vi "Init Controls.vi"(7 "connected":bool, 8 "Fehler (Eingang, kein Fehler)":errorcluster, 10 "Cluster Refernz Cluster":T1, 11 "Info Cluster":T2) -> (0 "Fehler (Ausgang)":errorcluster, 6 "connected out":bool)   [LabVIEW 2020, in "Linearisierung v2.lvlib" / "Gasteiler.lvlib" / "HovaCAL_Interface.lvlib" / "Helper.lvlib"]
uses:
  Helper.lvlib
  Controls/Info Cluster.ctl
  Controls/Controls.lvlib
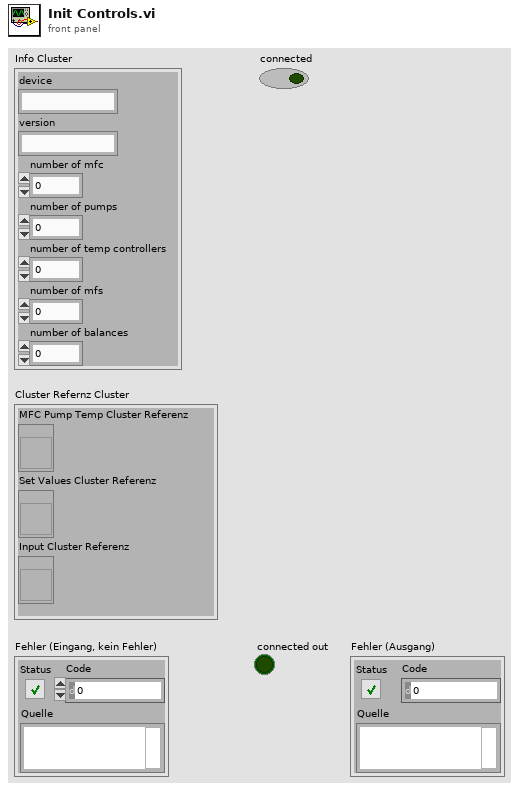
[diagram p1: front panel]
types:
  T1 = cluster{"MFC Pump Temp Cluster Referenz":refnum<vi>, "Set Values Cluster Referenz":refnum<vi>, "Input Cluster Referenz":refnum<vi>}
  T2 = typedef "Linearisierung v2.lvlib/Gasteiler.lvlib/HovaCAL_Interface.lvlib/Controls.lvlib/Info Cluster.ctl" = cluster{"device":string, "version":string, "number of mfc":i32, "number of pumps":i32, "number of temp controllers":i32, "number of mfs":i32, "number of balances":i32}
  T3 = enum8{"Enabled", "Disabled", "Disabled and Grayed Out"}
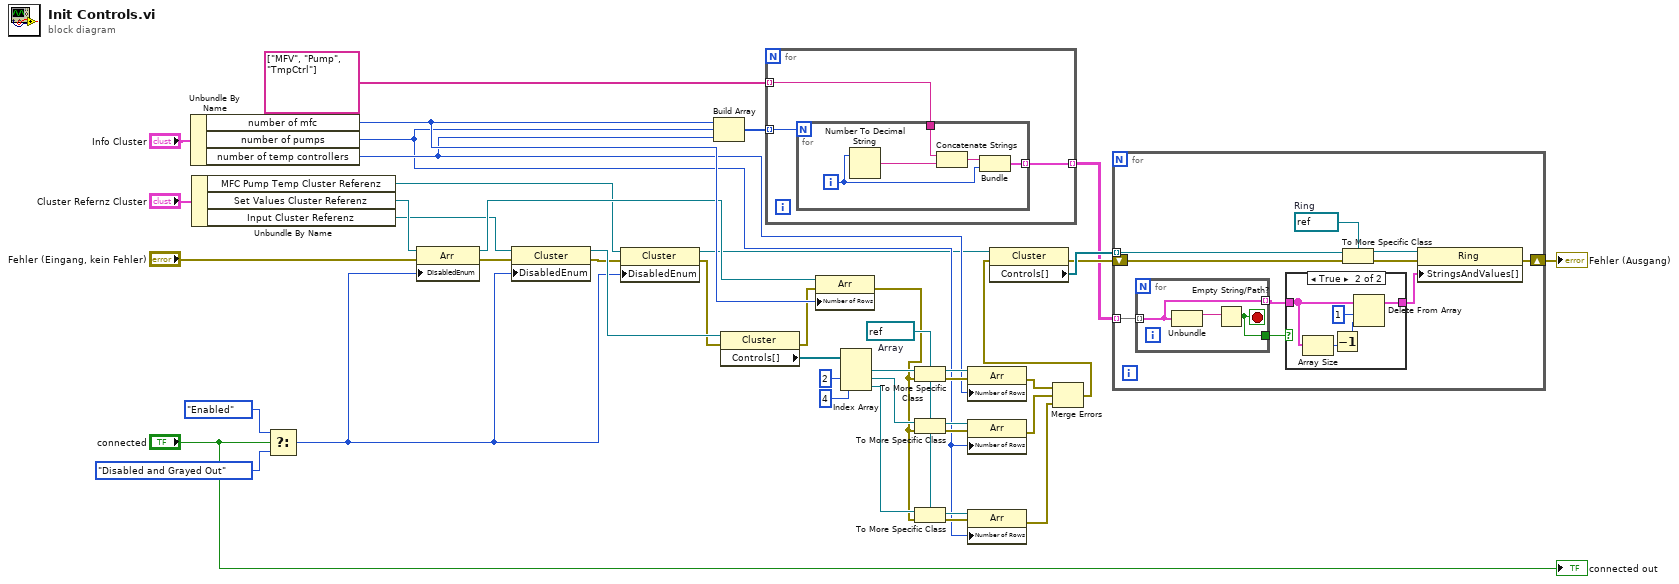
[diagram p0: block diagram]
diagram:
  w24 = refnum<vi> refnum  # Array
  n1 = Unbundle By Name("Info Cluster") -> ("number of mfc"=w36:i32, "number of pumps"=w15:i32, "number of temp controllers"=w16:i32)
  n2 = Unbundle By Name("Cluster Refernz Cluster") -> ("MFC Pump Temp Cluster Referenz"=w4:refnum<vi>, "Set Values Cluster Referenz"=w10:refnum<vi>, "Input Cluster Referenz"=w8:refnum<vi>)
  n3 = Select(t=T3."Enabled" ("Deaktiviert"), s="connected", f=T3."Disabled and Grayed Out" ("Deaktiviert")) -> (s? t:f=w2:T3)
  n4 = property class="Arr"(reference=w10, error in="Fehler (Eingang, kein Fehler)", "DisabledEnum"=w2) -> (reference out=w9:refnum<vi>, error out=w11:errorcluster)
  n5 = property class="Cluster"(reference=w8, error in=w11, "DisabledEnum"=w2) -> (reference out=w6:refnum<vi>, error out=w5:errorcluster)
  n6 = property class="Cluster"(reference=w4, error in=w5, "DisabledEnum"=w2) -> (reference out=w1:refnum<vi>, error out=w3:errorcluster)
  n7 = Build Array(w36, w15, w16) -> (w40:i32[])
  n8 = property class="Cluster"(reference=w6, error in=w3) -> (error out=w23:errorcluster, "Controls[]"=w35:refnum<vi>[])  [unwired: 1 out]
  n9 = for {
    tunnel: w40 -> [w47] mode=indexing
    tunnel: string[] ["MFV", "Pump", "TmpCtrl"] -> [w46] mode=indexing
    tunnel: [w45] -> w39 mode=indexing
    n10 = for {
      N: w47 -> [_]
      tunnel: [w52] -> w45 mode=indexing
      tunnel: w46 -> [w48]
      i -> [w51]
      n11 = Number To Decimal String(number=w51) -> (decimal integer string=w50:string)  [unwired: 1 in]
      n12 = Concatenate Strings(w48, w50) -> (w49:string)
      n13 = Bundle(w49, w51) -> (w52:cluster{string, i32})  [unwired: 1 in]
    }
  }
  n14 = property class="Arr"(reference=w9, error in=w23, "Number of Rows"=w36) -> (error out=w22:errorcluster)  [unwired: 1 out]
  n15 = Index Array(array=w35, index #2=2 ("Index"), index #3=4 ("Index")) -> (element #1=w32:refnum<vi>, element #2=w28:refnum<vi>, element #3=w25:refnum<vi>)  [unwired: 1 in]
  n16 = To More Specific Class(target class=w24, reference=w32, error in=w22) -> (specific class reference=w31:refnum<vi>, error out=w21:errorcluster)
  n17 = To More Specific Class(target class=w24, reference=w28, error in=w22) -> (specific class reference=w27:refnum<vi>, error out=w30:errorcluster)
  n18 = To More Specific Class(target class=w24, reference=w25, error in=w22) -> (specific class reference=w26:refnum<vi>, error out=w29:errorcluster)
  n19 = property class="Arr"(reference=w31, error in=w21, "Number of Rows"=w16) -> (error out=w20:errorcluster)  [unwired: 1 out]
  n20 = property class="Arr"(reference=w27, error in=w30, "Number of Rows"=w15) -> (error out=w19:errorcluster)  [unwired: 1 out]
  n21 = property class="Arr"(reference=w26, error in=w29, "Number of Rows"=w15) -> (error out=w18:errorcluster)  [unwired: 1 out]
  n22 = Merge Errors(w20, w19, w18) -> (w17:errorcluster)
  n23 = property class="Cluster"(reference=w1, error in=w17) -> (error out=w42:errorcluster, "Controls[]"=w43:refnum<vi>[])  [unwired: 1 out]
  n24 = for {
    tunnel: w43 -> [w62] mode=indexing
    tunnel: w39 -> [w56] mode=indexing
    shift-right: [w57] -> w38
    shift-left: w42 -> [w61]
    w58 = refnum<vi> refnum  # Ring
    n25 = for {
      tunnel: w56 -> [w70] mode=indexing
      tunnel: [w70] -> w54 mode=indexing
      tunnel: [w69] -> w55
      stop <- w69 stop-if-true
      n26 = Unbundle(w70) -> (w71:string)  [unwired: 1 out]
      n27 = Empty String/Path?(string/path=w71) -> (empty?=w69:bool)
    }
    n28 = case shown="True" w55 {
      tunnel: w54 -> [w63 w68]
      tunnel: [w63 w65] -> w53
      frame False {
      }
      frame True {
        n29 = Array Size(array=w68) -> (size(s)=w67:i32)
        n30 = Decrement(x=w67) -> (x-1=w64:i32)
        n31 = Delete From Array(array=w68, length=1 ("Länge"), index=w64) -> (array with subset deleted=w65:cluster{string, i32}[])  [unwired: 1 out]
      }
    }
    n32 = To More Specific Class(target class=w58, reference=w62, error in=w61) -> (specific class reference=w59:refnum<vi>, error out=w60:errorcluster)
    n33 = property class="Ring"(reference=w59, error in=w60, "StringsAndValues[]"=w53) -> (error out=w57:errorcluster)  [unwired: 1 out]
  }
  "Fehler (Ausgang)" <- w38
  "connected out" <- "connected"
